vi "SDT_ReadFileBlock.vi"(8 "error in":errorcluster, 9 "MeasureInfo":T7[](array[typedef]) {"MeasFCSInfo"."fcs_decay_calc" format="%x"; "MeasStopInfo"."flags" format="x%x"; "MeasureInfo_PartB"."mod_type2" format="%016x"; "MeasureInfo_PartB"."mod_type1" format="%016x"}, 10 "bhfile_header":T6 {"chksum" format="x%x"; "header_valid" format="x%x"}, 11 "SDTFileRefnum":refnum<file>) -> (0 "error out":errorcluster, 1 "DecayMatrix":cluster{"Waveform Graph":sgl[]}[][](array[cluster]), 2 "IntensityImage":cluster{"Intensity Graph":u8[][]}[](array[cluster]), 3 "BHFileBlockHeader_interpreted":T1[](array[typedef]) {"lblock_Contents" items=["DECAY_BLOCK"=0, "PAGE_BLOCK"=16, "FCS_BLOCK"=32, "FIDA_BLOCK"=48, "FILDA_BLOCK"=64, "MCS_BLOCK"=80, "IMG_BLOCK"=96, "MCST_BLOCK"=112, "IMG_MCS_BLOCK"=128, "MOM_BLOCK"=144, "IMG_INT_BLOCK"=160, "IMG_WF_BLOCK"=176, "IMG_LIFE_BLOCK"=192]; "CreationMode" items=["NOT_USED"=0, "MEAS_DATA"=1, "FLOW_DATA"=2, "MEAS_DATA_FROM_FILE"=3, "CALC_DATA"=4, "SIM_DATA"=5, "FIFO_DATA"=8, "FIFO_DATA_FROM_FILE"=9, "MOM_DATA"=10, "MOM_DATA_FROM_FILE"=11]; "Contents" items=["DECAY_BLOCK"=0, "PAGE_BLOCK"=16, "FCS_BLOCK"=32, "FIDA_BLOCK"=48, "FILDA_BLOCK"=64, "MCS_BLOCK"=80, "IMG_BLOCK"=96, "MCST_BLOCK"=112, "IMG_MCS_BLOCK"=128, "MOM_BLOCK"=144, "IMG_INT_BLOCK"=160, "IMG_WF_BLOCK"=176, "IMG_LIFE_BLOCK"=192]; "DataType" items=["DATA_USHORT (U16)"=0, "DATA_ULONG (U32)"=256, "DATA_DBL (DBL64)"=512]; "BHFileBlockHeader"."lblock_no" format="x%x"; "BHFileBlockHeader"."block_type" format="%x"}, 4 "FCS_Block":cluster{"XY Graph":cluster{dbl[], dbl[]}}[](array[cluster]), 5 "SumOfDecays":dbl[][](graph))   [LabVIEW 2023]
doc: "This VI is a SubVI to SDT_ReadFile.vi. It reads the BHFileBlockHeader and data blocks in a SDT-file from disc.\nFor a description of the *.sdt file format see: SPC_data_file_structure.h\n\ninfo@becker-hickl.com"
uses:
  SPC_Wrappers/SPC_Controls/MeasureInfo.ctl
  SPC_Wrappers/SPC_Controls/MeasureInfo_PartB.ctl
  SPC_Wrappers/SPC_Controls/MeasStopInfo.ctl
  SPC_Wrappers/SPC_Controls/MeasFCSInfo.ctl
  SPC_Wrappers/SPC_Controls/MeasureInfo_PartE.ctl
  SPC_Wrappers/SPC_Controls/MeasHISTInfo.ctl
  SPC_Wrappers/SPC_Controls/HISTInfoExt.ctl
  SPC_Wrappers/SPC_Controls/MeasureInfo_PartI.ctl
  SPC_Wrappers/SPC_Controls/MeasureInfo_PartK.ctl
  SPC_Wrappers/SPC_Controls/MeasureInfo_PartM.ctl
  SPC_Wrappers/SPC_Controls/bhfile_header.ctl
  SPC_Wrappers/SPC_Controls/BHFileBlockHeader_interpreted.ctl
  SPC_Wrappers/SPC_Controls/BHFileBlockHeader.ctl
  SPC_Wrappers/SPC_Controls/BlockType_DataType.ctl
  SPC_Wrappers/SPC_Controls/BlockType_Contents.ctl
  SPC_Wrappers/SPC_Controls/BlockType_CreationMode.ctl
panel:
  # "block_type"
  # "lblock_no"
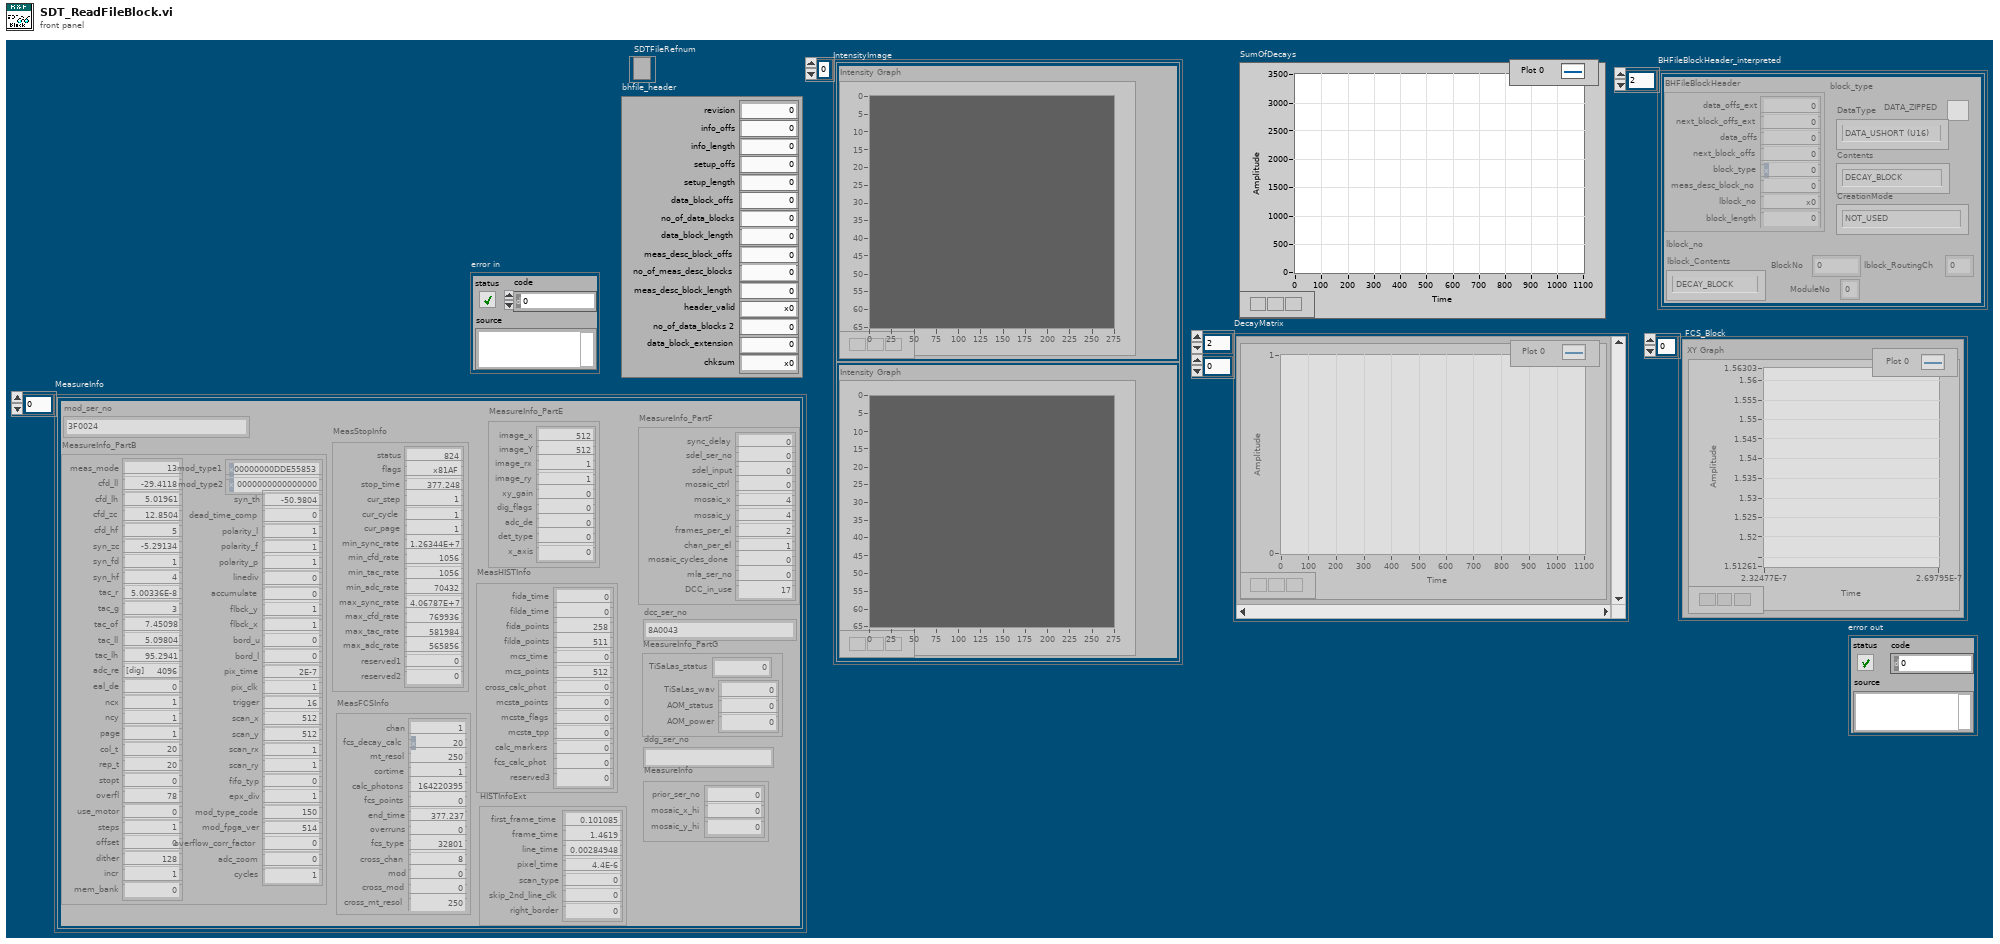
[diagram p1: front panel]
types:
  T1 = typedef "BHFileBlockHeader_interpreted.ctl" = cluster{"BHFileBlockHeader":T2, "DATA_ZIPPED":bool, "DataType":T3, "Contents":T4, "CreationMode":T5, "lblock_Contents":T4, "ModuleNo":u8, "BlockNo":u32, "lblock_RoutingCh":u32}
  T2 = typedef "BHFileBlockHeader.ctl" = cluster{"data_offs_ext":u8, "next_block_offs_ext":u8, "data_offs":u32, "next_block_offs":u32, "block_type":u16, "meas_desc_block_no":i16, "lblock_no":u32, "block_length":u32}
  T3 = typedef "BlockType_DataType.ctl" = u16
  T4 = typedef "BlockType_Contents.ctl" = u16
  T5 = typedef "BlockType_CreationMode.ctl" = u16
  T6 = typedef "bhfile_header.ctl" = cluster{"revision":i16, "info_offs":i32, "info_length":i16, "setup_offs":i32, "setup_length":u16, "data_block_offs":i32, "no_of_data_blocks":i16, "data_block_length":u32, "meas_desc_block_offs":i32, "no_of_meas_desc_blocks":i16, "meas_desc_block_length":i16, "header_valid":u16, "no_of_data_blocks 2":u32, "data_block_extension":u16, "chksum":u16}
  T7 = typedef "MeasureInfo.ctl" = cluster{"mod_ser_no":string, "MeasureInfo_PartB":T8, "MeasStopInfo":T9, "MeasFCSInfo":T10, "MeasureInfo_PartE":T11, "MeasHISTInfo":T12, "HISTInfoExt":T13, "MeasureInfo_PartF":T14, "dcc_ser_no":string, "MeasureInfo_PartG":T15, "ddg_ser_no":string, "MeasureInfo":T16}
  T8 = typedef "MeasureInfo_PartB.ctl" = cluster{"meas_mode":i16, "cfd_ll":sgl, "cfd_lh":sgl, "cfd_zc":sgl, "cfd_hf":sgl, "syn_zc":sgl, "syn_fd":i16, "syn_hf":sgl, "tac_r":sgl, "tac_g":i16, "tac_of":sgl, "tac_ll":sgl, "tac_lh":sgl, "adc_re":i16, "eal_de":i16, "ncx":i16, "ncy":i16, "page":u16, "col_t":sgl, "rep_t":sgl, "stopt":i16, "overfl":i8, "use_motor":i16, "steps":u16, "offset":sgl, "dither":i16, "incr":i16, "mem_bank":i16, "mod_type1":u64, "mod_type2":u64, "syn_th":sgl, "dead_time_comp":i16, "polarity_l":i16, "polarity_f":i16, "polarity_p":i16, "linediv":i16, "accumulate":i16, "flbck_y":i32, "flbck_x":i32, "bord_u":i32, "bord_l":i32, "pix_time":sgl, "pix_clk":i16, "trigger":i16, "scan_x":i32, "scan_y":i32, "scan_rx":i32, "scan_ry":i32, "fifo_typ":i16, "epx_div":i32, "mod_type_code":u16, "mod_fpga_ver":u16, "overflow_corr_factor":sgl, "adc_zoom":i32, "cycles":i32}
  T9 = typedef "MeasStopInfo.ctl" = cluster{"status":u16, "flags":u16, "stop_time":sgl, "cur_step":i32, "cur_cycle":i32, "cur_page":i32, "min_sync_rate":sgl, "min_cfd_rate":sgl, "min_tac_rate":sgl, "min_adc_rate":sgl, "max_sync_rate":sgl, "max_cfd_rate":sgl, "max_tac_rate":sgl, "max_adc_rate":sgl, "reserved1":i32, "reserved2":sgl}
  T10 = typedef "MeasFCSInfo.ctl" = cluster{"chan":u16, "fcs_decay_calc":u16, "mt_resol":u32, "cortime":sgl, "calc_photons":u32, "fcs_points":i32, "end_time":sgl, "overruns":u16, "fcs_type":u16, "cross_chan":u16, "mod":u16, "cross_mod":u16, "cross_mt_resol":u32}
  T11 = typedef "MeasureInfo_PartE.ctl" = cluster{"image_x":i32, "image_Y":i32, "image_rx":i32, "image_ry":i32, "xy_gain":i16, "dig_flags":i16, "adc_de":i16, "det_type":i16, "x_axis":i16}
  T12 = typedef "MeasHISTInfo.ctl" = cluster{"fida_time":sgl, "filda_time":sgl, "fida_points":i32, "filda_points":i32, "mcs_time":sgl, "mcs_points":i32, "cross_calc_phot":u32, "mcsta_points":u16, "mcsta_flags":u16, "mcsta_tpp":u32, "calc_markers":u32, "fcs_calc_phot":u32, "reserved3":u32}
  T13 = typedef "HISTInfoExt.ctl" = cluster{"first_frame_time":sgl, "frame_time":sgl, "line_time":sgl, "pixel_time":sgl, "scan_type":i16, "skip_2nd_line_clk":i16, "right_border":u32}
  T14 = typedef "MeasureInfo_PartI.ctl" = cluster{"sync_delay":sgl, "sdel_ser_no":u16, "sdel_input":i8, "mosaic_ctrl":i8, "mosaic_x":u8, "mosaic_y":u8, "frames_per_el":i16, "chan_per_el":i16, "mosaic_cycles_done":i32, "mla_ser_no":u16, "DCC_in_use":u8}
  T15 = typedef "MeasureInfo_PartK.ctl" = cluster{"TiSaLas_status":u16, "TiSaLas_wav":u16, "AOM_status":u8, "AOM_power":u8}
  T16 = typedef "MeasureInfo_PartM.ctl" = cluster{"prior_ser_no":i32, "mosaic_x_hi":u8, "mosaic_y_hi":u8}
  T17 = enum16{"big-endian, network order", "native, host order", "little-endian"}
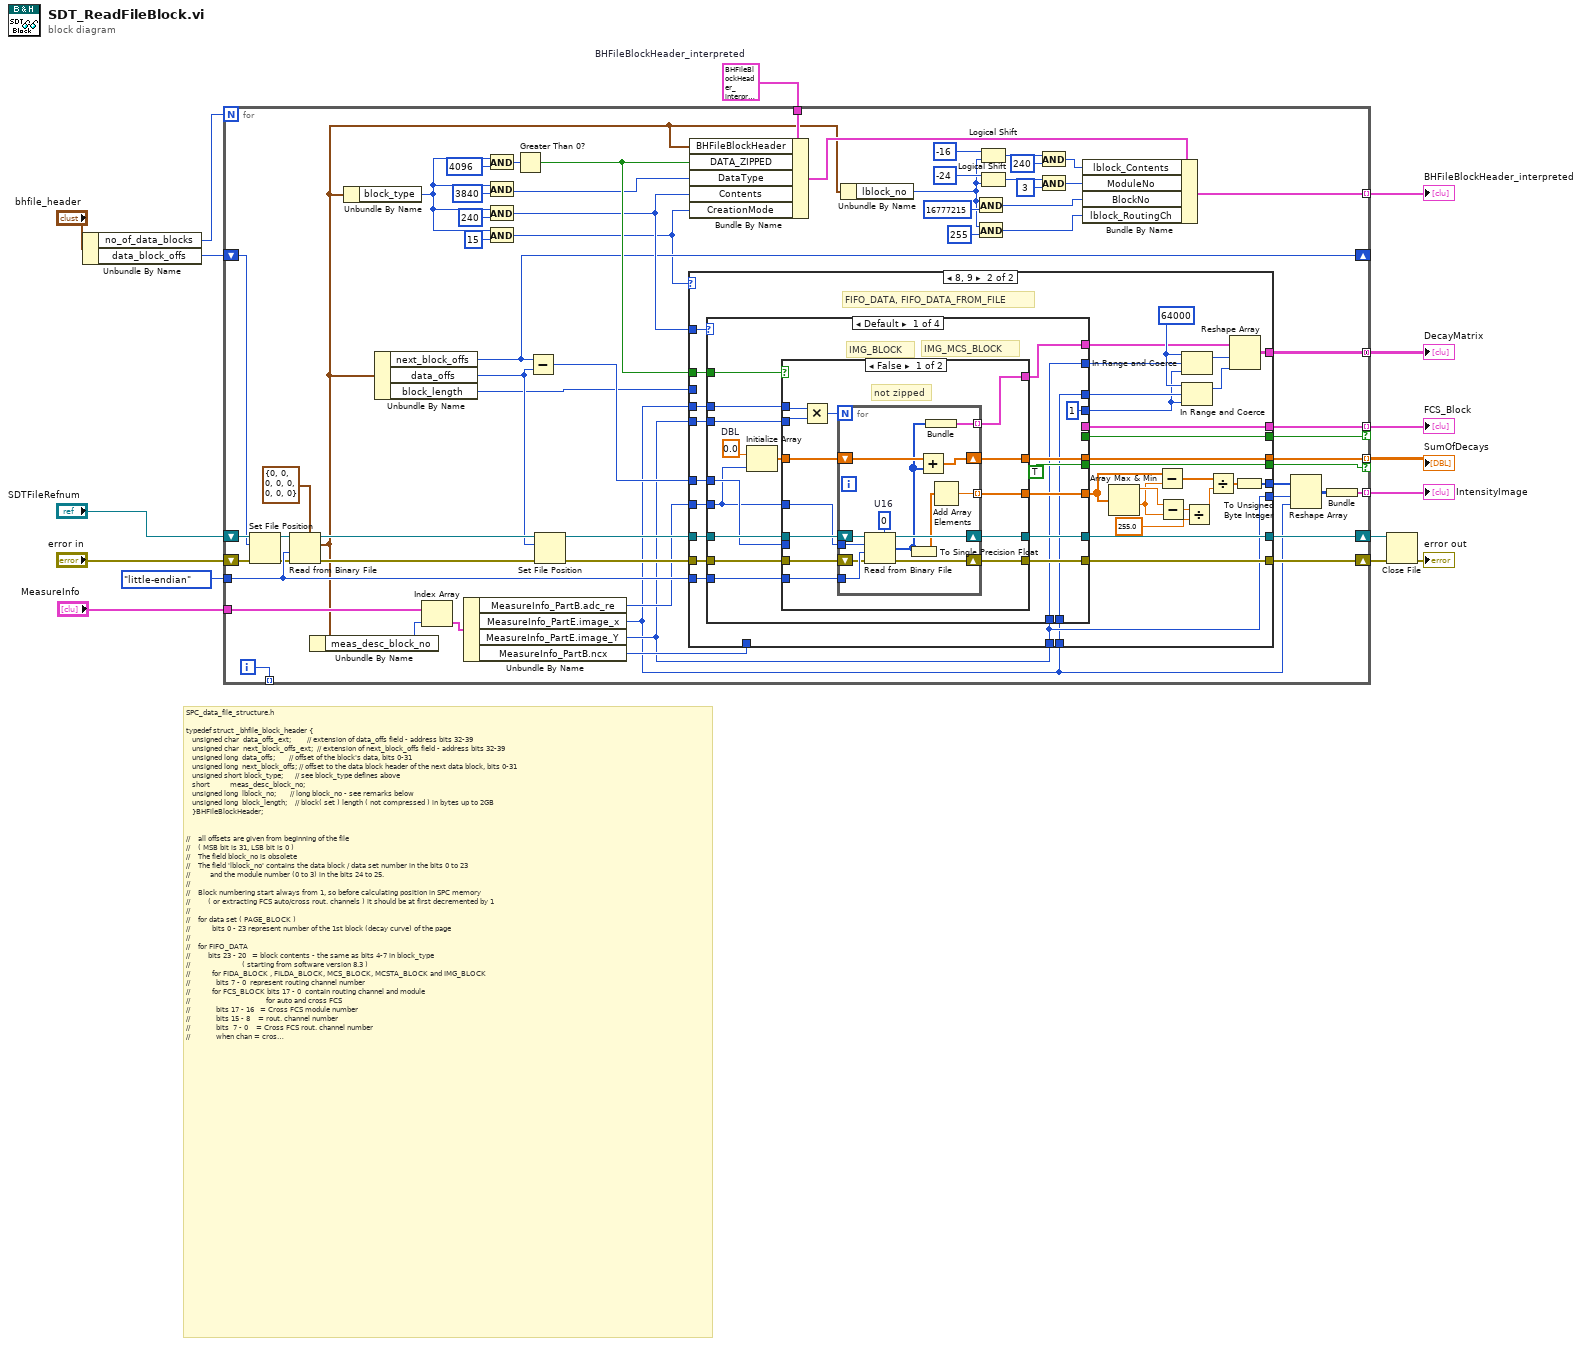
[diagram p0: block diagram]
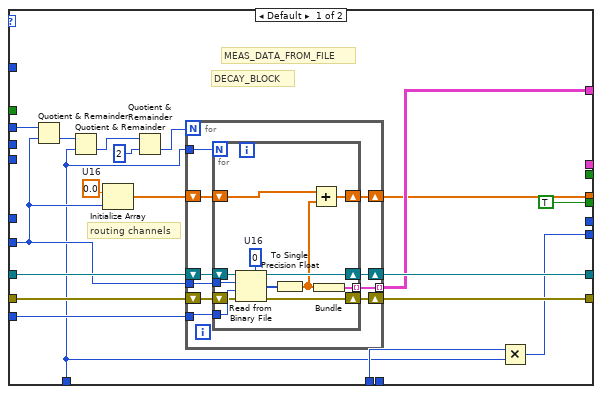
[diagram p2: hidden frame]
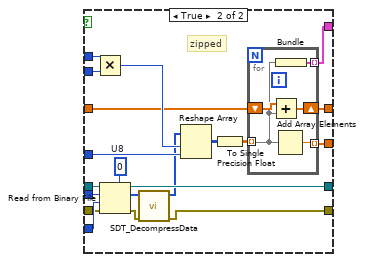
[diagram p3: hidden frame]
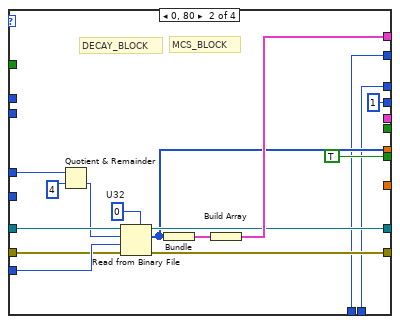
[diagram p4: hidden frame]
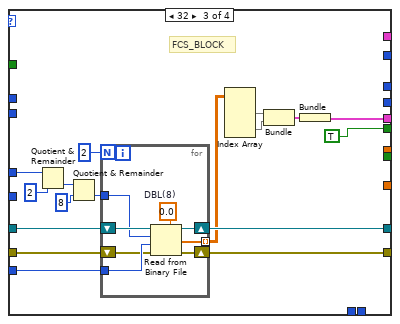
[diagram p5: hidden frame]
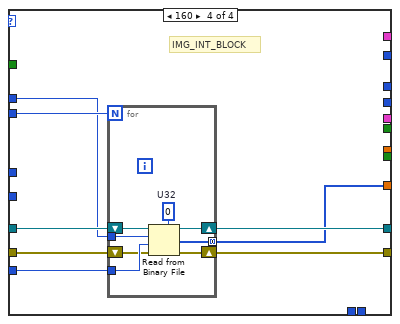
[diagram p6: hidden frame]
diagram:
  w3 = T1 {"BHFileBlockHeader"={"data_offs_ext"=0, "next_block_offs_ext"=0, "data_offs"=0, "next_block_offs"=0, "block_type"=0, "meas_desc_block_no"=0, "lblock_no"=0, "block_length"=0}, "DATA_ZIPPED"=FALSE, "DataType"=0, "Contents"=0, "CreationMode"=11, "lblock_Contents"=128, "ModuleNo"=0, "BlockNo"=0, "lblock_RoutingCh"=0}  # BHFileBlockHeader_interpreted
  # "SPC_data_file_structure.h\n\ntypedef struct _bhfile_block_header {\n   unsigned char  data_offs_ext;        // extension of data_offs field - address bits 32-39\n   unsigned char  next_block_offs_ext;  // extension of next_block_offs field - address bits 32-39\n   unsigned long  data_offs;       // offset of the block's data, bits 0-31  \n   unsigned long  next_block_offs; // offset to the data block header of the next data block, bits 0-31 \n   unsigned short block_type;      // see block_type defines above\n   short          meas_desc_block_no;\n   unsigned long  lblock_no;       // long block_no - see remarks below\n   unsigned long  block_length;    // block( set ) length ( not compressed ) in bytes up to 2GB\n   }BHFileBlockHeader;\n\n\n//    all offsets are given from beginning of the file\n//    ( MSB bit is 31, LSB bit is 0 )\n//    The field block_no is obsolete\n//    The field 'lblock_no' contains the data block / data set number in the bits 0 to 23 \n//          and the module number (0 to 3) in the bits 24 to 25.\n//\n//    Block numbering start always from 1, so before calculating position in SPC memory \n//         ( or extracting FCS auto/cross rout. channels ) it should be at first decremented by 1\n//    \n//    for data set ( PAGE_BLOCK ) \n//           bits 0 - 23 represent number of the 1st block (decay curve) of the page\n//\n//    for FIFO_DATA \n//         bits 23 - 20   = block contents - the same as bits 4-7 in block_type\n//                          ( starting from software version 8.3 )\n//           for FIDA_BLOCK , FILDA_BLOCK, MCS_BLOCK, MCSTA_BLOCK and IMG_BLOCK\n//             bits 7 - 0  represent routing channel number\n//           for FCS_BLOCK bits 17 - 0  contain routing channel and module \n//                                      for auto and cross FCS\n//             bits 17 - 16   = Cross FCS module number\n//             bits 15 - 8    = rout. channel number   \n//             bits  7 - 0    = Cross FCS rout. channel number   \n//             when chan = cross_chan and mod == cross_mod - Auto FCS, \n//                           otherwise - Cross FCS\n//    for MOM_DATA \n//         bits 23 - 20   = block(set) contents - the same as bits 4-7 in block_type\n//         bits 19 -  0   = number of the data set\nee"
  n1 = Unbundle By Name("bhfile_header") -> ("no_of_data_blocks"=w11:i16, "data_block_offs"=w12:i32)
  n2 = for {
    N: w11 -> [_]
    tunnel: T17."little-endian" ("byte order (0:big-endian, network order)") -> [w61]
    tunnel: [w62] -> w16 mode=indexing
    shift-right: [w28] -> _
    shift-left: w12 -> [w60]
    shift-right: [w59] -> w15
    shift-left: "SDTFileRefnum" -> [w65]
    tunnel: [w22] -> w14 mode=concatenating
    tunnel: [w57] -> w13 mode=indexing if=w18
    tunnel: [w56] -> _ mode=indexing
    tunnel: "MeasureInfo" -> [w52]
    shift-right: [w46] -> w10
    shift-left: "error in" -> [w50]
    tunnel: w3 -> [w45]
    tunnel: [w34] -> w2 mode=indexing
    tunnel: [w26] -> w1 mode=indexing if=w17
    i -> [w56]
    n3 = Set File Position(offset (in bytes) (0)=w60, refnum=w65, error in=w50) -> (refnum out=w63:refnum<file>, error out=w49:errorcluster)  [unwired: 1 in]
    n4 = Read from Binary File(5:T2 {"data_offs_ext"=0, "next_block_offs_ext"=0, "data_offs"=0, "next_block_offs"=0, "block_type"=0, "meas_desc_block_no"=0, "lblock_no"=0, "block_length"=0} ("BHFileBlockHeader"), 8:w49, 9:w61, 11:w63) -> (0:w48:errorcluster, 2:w30:T2, 3:w64:refnum<file>)  [unwired: 2 in, 1 out]
    n5 = Unbundle By Name(w30) -> ("meas_desc_block_no"=w29:i16)
    n6 = Unbundle By Name(w30) -> ("block_type"=w35:u16)
    n7 = Unbundle By Name(w30) -> ("next_block_offs"=w28:u32, "data_offs"=w27:u32, "block_length"=w25:u32)
    n8 = Index Array(array=w52, index=w29) -> (element=w51:T7)
    n9 = Unbundle By Name(w51) -> ("MeasureInfo_PartB.adc_re"=w31:i16, "MeasureInfo_PartE.image_x"=w20:i32, "MeasureInfo_PartE.image_Y"=w23:i32, "MeasureInfo_PartB.ncx"=w24:i16)
    n10 = And(x=w35, y=u16 4096) -> (x .and. y?=w72:u16)
    n11 = And(x=w35, y=u16 3840) -> (x .and. y?=w43:u16)
    n12 = And(x=w35, y=u16 240) -> (x .and. y?=w42:u16)
    n13 = And(x=w35, y=u16 15) -> (x .and. y?=w19:u16)
    n14 = Greater Than 0?(x=w72) -> (x > 0?=w44:bool)
    n15 = Subtract(x=w28, y=w27) -> (x-y=w58:u32)
    n16 = Set File Position(offset (in bytes) (0)=w27, refnum=w64, error in=w48) -> (refnum out=w67:refnum<file>, error out=w47:errorcluster)  [unwired: 1 in]
    n17 = case shown="8, 9" w19 {
      tunnel: w67 -> [w96 w152]
      tunnel: [w91 w151] -> w26
      tunnel: w44 -> [_ w150]
      tunnel: w61 -> [w95 w149]
      tunnel: [w94 w148] -> w59
      tunnel: w20 -> [_ w147]
      tunnel: w23 -> [_ w146]
      tunnel: w31 -> [w88 w145]
      tunnel: w58 -> [_ w144]
      tunnel: w25 -> [w93 _]
      tunnel: [w92 w128] -> w22
      tunnel: w42 -> [_ w143]
      tunnel: [_ w142] -> w57
      tunnel: w47 -> [w86 w141]
      tunnel: [w85 w140] -> w46
      tunnel: [_ w131] -> w32
      tunnel: w24 -> [w80 _]
      tunnel: [w81 w123] -> w21
      tunnel: w23 -> [w82 w123]
      tunnel: w20 -> [_ w121]
      tunnel: [_ w125] -> w18
      tunnel: [TRUE w124] -> w17
      frame Default {
        w89 = sgl 0.0  # U16
        # "routing channels"
        # "MEAS_DATA_FROM_FILE"
        # "DECAY_BLOCK"
        n18 = Quotient & Remainder(x=w93, y=w88) -> (floor(x/y)=w84:u32)  [unwired: 1 out]
        n19 = Quotient & Remainder(x=w84, y=w80) -> (floor(x/y)=w83:u32)  [unwired: 1 out]
        n20 = Initialize Array(w89, w88) -> (w87:sgl[])
        n21 = Quotient & Remainder(x=w83, y=u32 2) -> (floor(x/y)=w79:u32)  [unwired: 1 out]
        n22 = for {
          N: w79 -> [_]
          tunnel: w95 -> [w105]
          tunnel: [w103] -> w92 mode=indexing
          tunnel: w80 -> [w101]
          tunnel: w88 -> [w100]
          shift-right: [w104] -> w94
          shift-left: w96 -> [w106]
          shift-right: [w97] -> w85
          shift-left: w86 -> [w98]
          shift-right: [w102] -> w91
          shift-left: w87 -> [w99]
          n23 = for {
            N: w101 -> [_]
            tunnel: w105 -> [w117]
            shift-right: [w115] -> w104
            shift-left: w106 -> [w118]
            tunnel: w100 -> [w114]
            tunnel: [w113] -> w103 mode=indexing
            shift-right: [w112] -> w102
            shift-left: w99 -> [w111]
            shift-right: [w109] -> w97
            shift-left: w98 -> [w110]
            w116 = u16 0  # U16
            n24 = Read from Binary File(5:w116, 8:w110, 9:w117, 10:w114, 11:w118) -> (0:w109:errorcluster, 2:w108:u16[], 3:w115:refnum<file>)  [unwired: 1 in, 1 out]
            n25 = To Single Precision Float(number=w108) -> (single precision float=w107:sgl[])
            n26 = Add(x=w111, y=w107) -> (x+y=w112:sgl[])
            n27 = Bundle(w107) -> (w113:cluster{sgl[]})  [unwired: 1 in]
          }
        }
        n28 = Multiply(x=w82, y=w80) -> (x*y=w81:i32)
      }
      frame 8, 9 {
        w130 = 64000 ("upper limit")
        # "FIFO_DATA, FIFO_DATA_FROM_FILE"
        n29 = case shown="Default" w143 {
          tunnel: w152 -> [w171 w238 w255 w271]
          tunnel: [w170 w227 _ _] -> w151
          tunnel: w150 -> [w169 _ _ _]
          tunnel: w149 -> [w168 w237 w254 w270]
          tunnel: [w167 w233 w253 w269] -> w148
          tunnel: w147 -> [w166 _ _ w267]
          tunnel: w146 -> [w165 _ _ w268]
          tunnel: w145 -> [w162 _ _ _]
          tunnel: w144 -> [w164 w231 w252 _]
          tunnel: [w157 w234 _ _] -> w129
          tunnel: [_ _ w240 _] -> w142
          tunnel: w141 -> [w160 w229 w242 w266]
          tunnel: [w159 w228 w241 w265] -> w140
          tunnel: [w158 _ _ w264] -> w132
          tunnel: [_ _ TRUE _] -> w125
          tunnel: [TRUE TRUE _ _] -> w124
          tunnel: w123 -> [w155 w224 _ _]
          tunnel: [w155 w224 _ _] -> w122
          tunnel: w121 -> [w154 w225 _ _]
          tunnel: [w154 w225 _ _] -> w120
          tunnel: [1 ("lower limit") 1 ("lower limit") _ _] -> w119
          frame Default {
            w163 = 0.0  # DBL
            # "IMG_MCS_BLOCK"
            # "IMG_BLOCK"
            n30 = Initialize Array(w163, w162) -> (w161:dbl[])
            n31 = case shown="False" w169 {
              tunnel: w171 -> [w184 w217]
              tunnel: [w183 w209] -> w158
              tunnel: [w181 w216] -> w167
              tunnel: [w176 w210] -> w170
              tunnel: w168 -> [w180 w203]
              tunnel: w166 -> [w178 w215]
              tunnel: w165 -> [w177 w214]
              tunnel: w162 -> [w179 w211]
              tunnel: w164 -> [_ w207]
              tunnel: w161 -> [w175 w202]
              tunnel: w160 -> [w174 w201]
              tunnel: [w173 w199] -> w159
              tunnel: [w172 w198] -> w157
              frame False {
                # "not zipped"
                n32 = Multiply(x=w178, y=w177) -> (x*y=w182:i32)
                n33 = for {
                  N: w182 -> [_]
                  tunnel: w180 -> [w196]
                  shift-right: [w194] -> w181
                  shift-left: w184 -> [w197]
                  tunnel: [w193] -> w183 mode=indexing
                  tunnel: w179 -> [w192]
                  shift-right: [w190] -> w176
                  shift-left: w175 -> [w189]
                  shift-right: [w187] -> w173
                  shift-left: w174 -> [w188]
                  tunnel: [w185] -> w172 mode=indexing
                  w195 = u16 0  # U16
                  n34 = Read from Binary File(5:w195, 8:w188, 9:w196, 10:w192, 11:w197) -> (0:w187:errorcluster, 2:w186:u16[], 3:w194:refnum<file>)  [unwired: 1 in, 1 out]
                  n35 = To Single Precision Float(number=w186) -> (single precision float=w191:sgl[])
                  n36 = Add(x=w189, y=w186) -> (x+y=w190:dbl[])
                  n37 = Bundle(w186) -> (w185:cluster{u16[]})  [unwired: 1 in]
                  n38 = Add Array Elements(numeric array=w191) -> (sum=w193:sgl)
                }
              }
              frame True {
                w204 = u8 0  # U8
                # "zipped"
                n39 = Multiply(x=w215, y=w214) -> (x*y=w212:i32)
                n40 = Read from Binary File(5:w204, 8:w201, 9:w203, 10:w207, 11:w217) -> (0:w200:errorcluster, 2:w208:u8[], 3:w216:refnum<file>)  [unwired: 1 in, 1 out]
                n41 = call "SDT_DecompressData.vi"("ErrorIn"=w200, "CompressedData"=w208) -> ("ErrorOut"=w199:errorcluster, "DecompressedData(U16)"=w205:u16[])  [unwired: 8 in]
                n42 = Reshape Array(w205, w212, w211) -> (w213:u16[][])
                n43 = To Single Precision Float(number=w213) -> (single precision float=w206:sgl[][])
                n44 = for {
                  tunnel: w206 -> [w219] mode=indexing
                  tunnel: [w222] -> w209 mode=indexing
                  shift-right: [w221] -> w210
                  shift-left: w202 -> [w220]
                  tunnel: [w218] -> w198 mode=indexing
                  n45 = Add(x=w220, y=w219) -> (x+y=w221:dbl[])
                  n46 = Add Array Elements(numeric array=w219) -> (sum=w222:sgl)
                  n47 = Bundle(w219) -> (w218:cluster{sgl[]})  [unwired: 1 in]
                }
              }
            }
          }
          frame 0, 80 {
            w236 = u32 0  # U32
            # "DECAY_BLOCK"
            # "MCS_BLOCK"
            n48 = Quotient & Remainder(x=w231, y=u32 4) -> (floor(x/y)=w232:u32)  [unwired: 1 out]
            n49 = Read from Binary File(5:w236, 8:w229, 9:w237, 10:w232, 11:w238) -> (0:w228:errorcluster, 2:w227:u32[], 3:w233:refnum<file>)  [unwired: 1 in, 1 out]
            n50 = Bundle(w227) -> (w235:cluster{u32[]})  [unwired: 1 in]
            n51 = Build Array(w235) -> (w234:cluster{u32[]}[])
          }
          frame 32 {
            # "FCS_BLOCK"
            n52 = Quotient & Remainder(x=w252, y=u32 2) -> (floor(x/y)=w245:u32)  [unwired: 1 out]
            n53 = Quotient & Remainder(x=w245, y=u32 8) -> (floor(x/y)=w244:u32)  [unwired: 1 out]
            n54 = for {
              N: 2 -> [_]
              tunnel: w254 -> [w262]
              tunnel: w244 -> [w259]
              tunnel: [w258] -> w249 mode=indexing
              shift-right: [w260] -> w253
              shift-left: w255 -> [w263]
              shift-right: [w256] -> w241
              shift-left: w242 -> [w257]
              w261 = 0.0  # DBL(8)
              n55 = Read from Binary File(5:w261, 8:w257, 9:w262, 10:w259, 11:w263) -> (0:w256:errorcluster, 2:w258:dbl[], 3:w260:refnum<file>)  [unwired: 1 in, 1 out]
            }
            n56 = Index Array(array=w249) -> (element #1=w248:dbl[], element #2=w247:dbl[])  [unwired: 4 in]
            n57 = Bundle(w248, w247) -> (w246:cluster{dbl[], dbl[]})  [unwired: 1 in]
            n58 = Bundle(w246) -> (w240:cluster{cluster{dbl[], dbl[]}})  [unwired: 1 in]
          }
          frame 160 {
            # "IMG_INT_BLOCK"
            n59 = for {
              N: w268 -> [_]
              tunnel: w270 -> [w278]
              tunnel: w267 -> [w275]
              tunnel: [w274] -> w264 mode=concatenating
              shift-right: [w276] -> w269
              shift-left: w271 -> [w279]
              shift-right: [w272] -> w265
              shift-left: w266 -> [w273]
              w277 = u32 0  # U32
              n60 = Read from Binary File(5:w277, 8:w273, 9:w278, 10:w275, 11:w279) -> (0:w272:errorcluster, 2:w274:u32[], 3:w276:refnum<file>)  [unwired: 1 in, 1 out]
            }
          }
        }
        n61 = Array Max & Min(array=w132) -> (max value=w139:sgl, min value=w138:sgl)  [unwired: 2 out]
        n62 = Subtract(x=w132, y=w138) -> (x-y=w135:sgl[])
        n63 = Subtract(x=w139, y=w138) -> (x-y=w137:sgl)
        n64 = In Range and Coerce(upper limit=w130, x=w122, lower limit=w119) -> (coerced(x)=w127:i32)  [unwired: 1 out]
        n65 = In Range and Coerce(upper limit=w130, x=w120, lower limit=w119) -> (coerced(x)=w126:i32)  [unwired: 1 out]
        n66 = Divide(x=w137, y=sgl 255.0 ("x")) -> (x/y=w133:sgl)
        n67 = Divide(x=w135, y=w133) -> (x/y=w134:sgl[])
        n68 = Reshape Array(w129, w127, w126) -> (w128:cluster{sgl[]}[][])
        n69 = To Unsigned Byte Integer(number=w134) -> (unsigned 8bit integer=w131:u8[])
      }
    }
    n70 = Bundle By Name(cluster=w45, "BHFileBlockHeader"=w30, "DATA_ZIPPED"=w44, "DataType"=w43, "Contents"=w42, "CreationMode"=w19) -> (w40:T1)
    n71 = Unbundle By Name(w30) -> ("lblock_no"=w41:u32)
    n72 = And(x=w41, y=u32 16777215) -> (x .and. y?=w37:u32)
    n73 = And(x=w41, y=u32 255) -> (x .and. y?=w36:u32)
    n74 = Logical Shift(y=i16 -16, x=w41) -> (x << y=w54:u32)
    n75 = Logical Shift(y=i16 -24, x=w41) -> (x << y=w70:u32)
    n76 = And(x=w54, y=i16 240) -> (x .and. y?=w39:u32)
    n77 = And(x=w70, y=i16 3) -> (x .and. y?=w38:u32)
    n78 = Bundle By Name(cluster=w40, "lblock_Contents"=w39, "ModuleNo"=w38, "BlockNo"=w37, "lblock_RoutingCh"=w36) -> (w34:T1)
    n79 = Reshape Array(w32, w21, w20) -> (w66:u8[][])
    n80 = Bundle(w66) -> (w62:cluster{u8[][]})  [unwired: 1 in]
  }
  "DecayMatrix" <- w14
  "FCS_Block" <- w13
  "IntensityImage" <- w16
  "BHFileBlockHeader_interpreted" <- w2
  "SumOfDecays" <- w1
  n81 = Close File(refnum=w15, error in=w10) -> (error out=→"error out":errorcluster)  [unwired: 1 out]
